vi "ALTS-2015 Get_ErrorString.vi"(8 "error in (no error)":errorcluster, 11 "Incoming Error":errorcluster) -> (0 "error out":errorcluster, 3 "Message":string)   [LabVIEW 2013]
uses:
  <vilib>/Utility/error.llb/DialogType.ctl
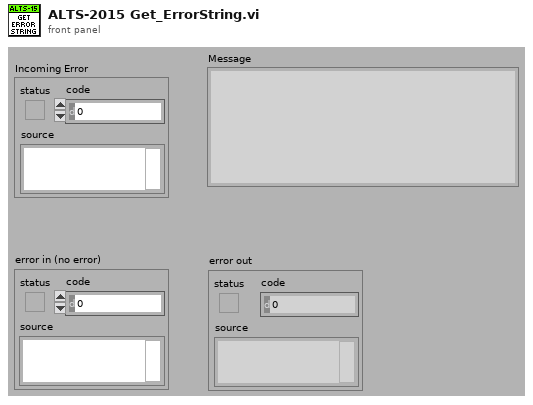
[diagram p1: front panel]
types:
  T1 = typedef "DialogType.ctl" = u16
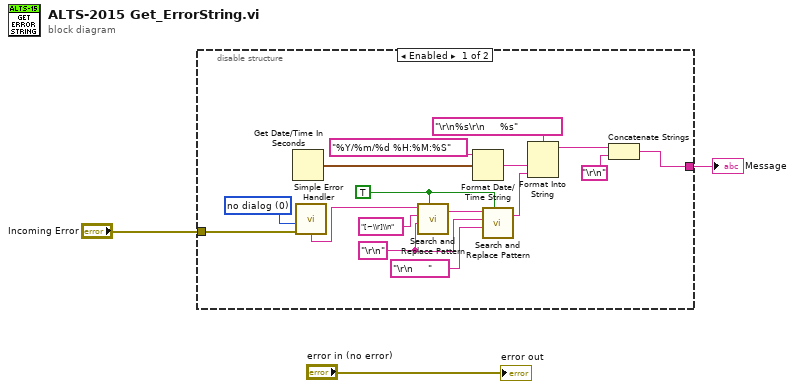
[diagram p0: block diagram]
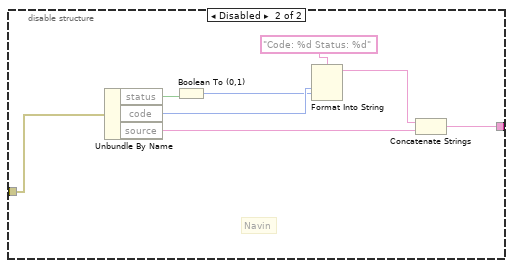
[diagram p2: hidden frame]
diagram:
  n1 = disable-structure shown="Enabled" {
    disable-tunnel: "Incoming Error" -> [w5 w27]
    disable-tunnel: [w4 w25] -> w2
    frame Enabled {
      w11 = "\r\n" ("regular expression (\"\")")
      w13 = TRUE ("replace all? (F)")
      w16 = T1 0 items=["no dialog", "OK message", "continue or stop message", "OK message + warnings", "continue/stop + warnings"] ("type of dialog (OK msg:1)")
      n2 = Get Date/Time In Seconds() -> (seconds since 1Jan1904=w7:timestamp)
      n3 = call <vilib>:"Simple Error Handler.vi"("type of dialog (OK msg:1)"=w16, "error in (no error)"=w5) -> ("message"=w15:string)  [unwired: 7 out]
      n4 = call <vilib>:"Search and Replace Pattern.vi"("string"=w15, "regular expression (\"\")"="[~\\r]\\n" ("regular expression (\"\")"), "replace string (\"\")"=w11, "replace all? (F)"=w13) -> ("result string"=w12:string)  [unwired: 2 out]
      n5 = Format Date/Time String(time format string (%c)="%Y/%m/%d %H:%M:%S", seconds (now)=w7) -> (date/time string=w8:string)  [unwired: 1 out]
      n6 = call <vilib>:"Search and Replace Pattern.vi"("string"=w12, "regular expression (\"\")"=w11, "replace string (\"\")"="\r\n     " ("regular expression (\"\")"), "replace all? (F)"=w13) -> ("result string"=w9:string)  [unwired: 2 out]
      n7 = Format Into String(format string="\r\n%s\r\n     %s", w8, w9) -> (resulting string=w18:string)  [unwired: 2 in, 1 out]
      n8 = Concatenate Strings(w18, "\r\n") -> (w4:string)
    }
    frame Disabled {
      # "Navin"
      n9 = Unbundle By Name(w27) -> ("status"=w21:bool, "code"=w22:i32, "source"=w26:string)
      n10 = Boolean To (0,1)(Boolean=w21) -> (0, 1=w20:i16)
      n11 = Format Into String(format string="Code: %d Status: %d", w22, w20) -> (resulting string=w24:string)  [unwired: 2 in, 1 out]
      n12 = Concatenate Strings(w24, w26) -> (w25:string)
    }
  }
  "Message" <- w2
  "error out" <- "error in (no error)"
